vi "Simple Parse State Queue.vi"(0 "State Queue":string, 7 "error in (no error)":errorcluster) -> (4 "Remain States":string, 8 "Next State":string)   [LabVIEW 2016, in "斯坦道总磷.lvlib"]
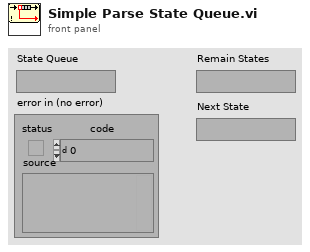
[diagram p1: front panel]
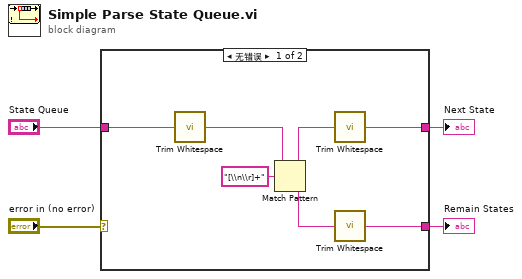
[diagram p0: block diagram]
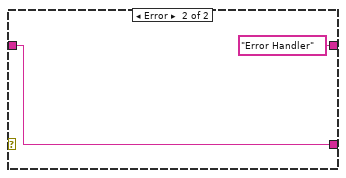
[diagram p2: hidden frame]
diagram:
  n1 = case shown="无错误" "error in (no error)" {
    tunnel: "State Queue" -> [w11 w13]
    tunnel: [w5 w13] -> w2
    tunnel: [w6 "Error Handler" ("State Queue")] -> w1
    frame No Error {
      n2 = call <vilib>:"Trim Whitespace.vi"("string"=w11) -> ("trimmed string"=w7:string)  [unwired: 1 in]
      n3 = Match Pattern(string=w7, regular expression="[\\n\\r]+") -> (before substring=w10:string, after substring=w9:string)  [unwired: 1 in, 2 out]
      n4 = call <vilib>:"Trim Whitespace.vi"("string"=w10) -> ("trimmed string"=w6:string)  [unwired: 1 in]
      n5 = call <vilib>:"Trim Whitespace.vi"("string"=w9) -> ("trimmed string"=w5:string)  [unwired: 1 in]
    }
    frame Error {
    }
  }
  "Remain States" <- w2
  "Next State" <- w1
